vi "FROG_RetrieveSignal.vi"(3 "Signal Template":cluster{"Gaussian noise pattern":dbl[], ext[]}, 5 "Traced Pulse":cdb[][](array[numeric])) -> (2 "Retrieved Signal":cluster{"Gaussian noise pattern":dbl[], ext[]})   [LabVIEW 2013]
uses:
  <vilib>/Analysis/baseanly.llb/Quick Scale 1D.vi
  <vilib>/Analysis/NI_AALBase.lvlib
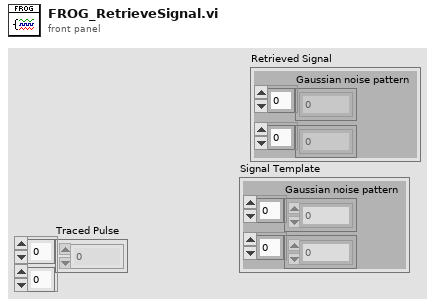
[diagram p1: front panel]
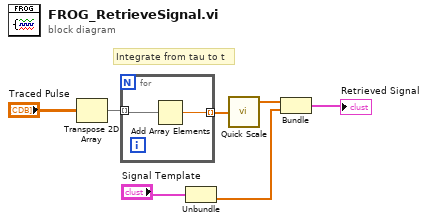
[diagram p0: block diagram]
diagram:
  # "Integrate from tau to t"
  n1 = Transpose 2D Array(2D array="Traced Pulse") -> (transposed array=w7:cdb[][])
  n2 = for {
    tunnel: w7 -> [w9] mode=indexing
    tunnel: [w8] -> w2 mode=indexing
    n3 = Add Array Elements(numeric array=w9) -> (sum=w8:cdb)
  }
  n4 = Unbundle("Signal Template") -> (w3:ext[])  [unwired: 1 out]
  n5 = call-poly <vilib>:"Quick Scale.vi"("X"=w2) -> ("Y[i]=X[i]/Max|X|"=w1:dbl[])  [unwired: 2 out]
  n6 = Bundle("Y[i]=X[i]/Max|X|"=w1, w3) -> (→"Retrieved Signal":cluster{"Y[i]=X[i]/Max|X|":dbl[], ext[]})  [unwired: 1 in]
